vi "swap test item name.vi"(11 "Diff Test Item Name":string[](array[string])) -> (3 "swapped test item name":string[](array[string]))   [LabVIEW 2011]
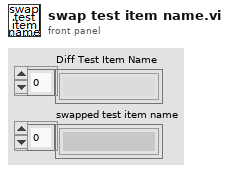
[diagram p1: front panel]
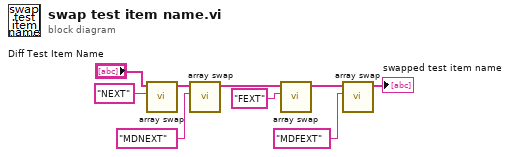
[diagram p0: block diagram]
diagram:
  n1 = call "array swap.vi"("search value"="NEXT", "array"="Diff Test Item Name") -> ("swapped array"=w5:string[])  [unwired: 9 in]
  n2 = call "array swap.vi"("search value"="MDNEXT", "array"=w5) -> ("swapped array"=w2:string[])  [unwired: 9 in]
  n3 = call "array swap.vi"("search value"="FEXT" ("元素"), "array"=w2) -> ("swapped array"=w7:string[])  [unwired: 9 in]
  n4 = call "array swap.vi"("search value"="MDFEXT", "array"=w7) -> ("swapped array"=→"swapped test item name":string[])  [unwired: 9 in]
